vi "GetAndWriteSlowCtrl.vi"(0 "queue in":T11, 1 "notifier in":T10, 2 "Data In":T1={"DAQ Config Data"={"Vertical"={"Coupling"=1, "Offset (V)"=-0.5, "Range (V)"=2.0, "Impedance"=50.0}, "Horizontal"={"Offset Time"=0.0, "Sample Time (S)"=22.0, "Sample Points"=1000}, "Trigger\n"={"Lower Level (V)"=-0.02, "Trigger Slope"=1, "Trigger Source"=10}, "Acquisition"={"Trigger Mode"=1, "Initiate Continuously"=0, "Acquire Type"=0, "Acquire Count"=1}, "Channel"=0, "Instrument Handle"=0, "Error"={"status"=FALSE, "code"=0, "source"=""}, "State"=1}, "Acquisition"={"Current"={"Acquiring Now?"=FALSE, "Waveforms Acquired"=0.0, "Start of Acquisition"=timestamp(0 s since 1904-01-01), "Acquisition Name"=""}, "Stop Condition"={"Quota"=3000.0, "Duration (S)"=22, "Stop Condition"=FALSE}, "Config Needed"=FALSE}, "Measurement"={"Waveform"={"t0"=timestamp(0 s since 1904-01-01), "dt"=1.0, "Y"=[]}, "Peak Heights"=[], "Acquisition Time"=timestamp(0 s since 1904-01-01), "File Path"=path "C:/Users/lab-341/Desktop/Reed/Oscilloscope VI/pulses.tdms", "TDMS File Handle"=refnum}, "UI References"={"Acquire"=refnum, "Configure DAQ"=refnum, "Measurement (Ch1)"=refnum, "Update Needed?"=FALSE, "New Run"=refnum, "Signal"=refnum}, "Run Info"={"Active Run?"=FALSE, "Run Notes"="Enter in notes explaining the purpose of the run and any unusual steps taken in the process. This should make it clear why the data was taken. e.g. \"Measuring LXe scintillation light with Teflon\" or \"Measuring dark pulses to determine SPE gain.\" Concise is good but precise is better.", "User Name"="", "Campaign ID#"="", "Run Name"="", "Start Time"=timestamp(0 s since 1904-01-01), "End Time"=timestamp(0 s since 1904-01-01)}, "System Status"={"Bias Voltage"=0.0, "SiPM Temperature"=[], "Slow Control User"="", "LXe"=0.0}, "Acquisition Info"={"Trigger Mode"=FALSE, "Acquisition Mode"=FALSE, "Bias Voltage (V)"=0.0, "Preamplifier"=0, "Shaping Amplifier"=0, "Acquisition Notes"="", "1"=FALSE, "2"=FALSE}} {"Acquisition Info"."Shaping Amplifier" items=["CR-200-100ns", "CR-200-1us"]; "Acquisition Info"."Preamplifier" items=["CR-Z-113-1k", "CR-Z-113-5k", "CR-Z-SiPM"]; "DAQ Config Data"."State" items=["Enable"=1, "Disable"=0]; "DAQ Config Data"."Channel" items=["Input Channel 1", "Input Channel 2", "Input Channel 3", "Input Channel 4"]; "DAQ Config Data"."Acquisition"."Acquire Type" items=["Normal"=0, "Average"=1, "Envelope"=2, "Peak Detect"=3, "High Resolution"=4, "Fast"=5, "Equivalent Time"=16]; "DAQ Config Data"."Acquisition"."Initiate Continuously" items=["Continuously"=1, "Single Capture"=0]; "DAQ Config Data"."Acquisition"."Trigger Mode" items=["Auto", "Normal"]; "DAQ Config Data"."Trigger"."Trigger Source" items=["TTL0", "TTL1", "TTL2", "TTL3", "TTL4", "TTL5", "TTL6", "TTL7", "ECL0", "ECL1", "Input Channel 1", "Input Channel 2", "Input Channel 3", "Input Channel 4", "External Trigger Source", "STAR", "Manual Trigger", "Pattern"]; "DAQ Config Data"."Trigger"."Trigger Slope" items=["Rising Edge", "Falling Edge"]; "DAQ Config Data"."Horizontal"."Sample Time (S)" items=["0.5"=0.5, "0.4"=0.4, "0.25"=0.25, "0.2"=0.2, "0.1"=0.1, "0.05"=0.05, "0.04"=0.04, "0.025"=0.025, "0.02"=0.02, "0.01"=0.01, "0.005"=0.005, "0.004"=0.004, "0.0025"=0.0025, "0.002"=0.002, "0.001"=0.001, "5E-4"=0.0005, "4E-4"=0.0004, "2.5E-4"=0.00025, "2E-4"=0.0002, "1E-4"=0.0001, "5E-5"=5e-05, "4E-5"=4e-05, "2E-5"=2e-05, "5E-6"=5e-06, "1E-6"=1e-06, "5E-7"=5e-07, "1E-7"=1e-07, "5E-8"=5e-08, "1E-8"=1e-08]; "DAQ Config Data"."Vertical"."Impedance" items=["50 Ohm"=50.0, "1 MOhm"=1000000.0]; "DAQ Config Data"."Vertical"."Range (V)" items=["10"=10.0, "5"=5.0, "2"=2.0, "1"=1.0, "0.4"=0.4, "0.2"=0.2, "0.08"=0.08, "0.04"=0.04, "0.02"=0.02, "0.01"=0.01]; "DAQ Config Data"."Vertical"."Coupling" items=["AC", "DC"]}) -> (7 "queue out":T11, 8 "notifier out":T10, 9 "Data Out":T1={"DAQ Config Data"={"Vertical"={"Coupling"=1, "Offset (V)"=-0.5, "Range (V)"=2.0, "Impedance"=50.0}, "Horizontal"={"Offset Time"=0.0, "Sample Time (S)"=22.0, "Sample Points"=1000}, "Trigger\n"={"Lower Level (V)"=-0.02, "Trigger Slope"=1, "Trigger Source"=10}, "Acquisition"={"Trigger Mode"=1, "Initiate Continuously"=0, "Acquire Type"=0, "Acquire Count"=1}, "Channel"=0, "Instrument Handle"=0, "Error"={"status"=FALSE, "code"=0, "source"=""}, "State"=1}, "Acquisition"={"Current"={"Acquiring Now?"=FALSE, "Waveforms Acquired"=0.0, "Start of Acquisition"=timestamp(0 s since 1904-01-01), "Acquisition Name"=""}, "Stop Condition"={"Quota"=3000.0, "Duration (S)"=22, "Stop Condition"=FALSE}, "Config Needed"=FALSE}, "Measurement"={"Waveform"={"t0"=timestamp(0 s since 1904-01-01), "dt"=1.0, "Y"=[]}, "Peak Heights"=[], "Acquisition Time"=timestamp(0 s since 1904-01-01), "File Path"=path "C:/Users/lab-341/Desktop/Reed/Oscilloscope VI/pulses.tdms", "TDMS File Handle"=refnum}, "UI References"={"Acquire"=refnum, "Configure DAQ"=refnum, "Measurement (Ch1)"=refnum, "Update Needed?"=FALSE, "New Run"=refnum, "Signal"=refnum}, "Run Info"={"Active Run?"=FALSE, "Run Notes"="Enter in notes explaining the purpose of the run and any unusual steps taken in the process. This should make it clear why the data was taken. e.g. \"Measuring LXe scintillation light with Teflon\" or \"Measuring dark pulses to determine SPE gain.\" Concise is good but precise is better.", "User Name"="", "Campaign ID#"="", "Run Name"="", "Start Time"=timestamp(0 s since 1904-01-01), "End Time"=timestamp(0 s since 1904-01-01)}, "System Status"={"Bias Voltage"=0.0, "SiPM Temperature"=[], "Slow Control User"="", "LXe"=0.0}, "Acquisition Info"={"Trigger Mode"=FALSE, "Acquisition Mode"=FALSE, "Bias Voltage (V)"=0.0, "Preamplifier"=0, "Shaping Amplifier"=0, "Acquisition Notes"="", "1"=FALSE, "2"=FALSE}} {"Acquisition Info"."Shaping Amplifier" items=["CR-200-100ns", "CR-200-1us"]; "Acquisition Info"."Preamplifier" items=["CR-Z-113-1k", "CR-Z-113-5k", "CR-Z-SiPM"]; "DAQ Config Data"."State" items=["Enable"=1, "Disable"=0]; "DAQ Config Data"."Channel" items=["Input Channel 1", "Input Channel 2", "Input Channel 3", "Input Channel 4"]; "DAQ Config Data"."Acquisition"."Acquire Type" items=["Normal"=0, "Average"=1, "Envelope"=2, "Peak Detect"=3, "High Resolution"=4, "Fast"=5, "Equivalent Time"=16]; "DAQ Config Data"."Acquisition"."Initiate Continuously" items=["Continuously"=1, "Single Capture"=0]; "DAQ Config Data"."Acquisition"."Trigger Mode" items=["Auto", "Normal"]; "DAQ Config Data"."Trigger"."Trigger Source" items=["TTL0", "TTL1", "TTL2", "TTL3", "TTL4", "TTL5", "TTL6", "TTL7", "ECL0", "ECL1", "Input Channel 1", "Input Channel 2", "Input Channel 3", "Input Channel 4", "External Trigger Source", "STAR", "Manual Trigger", "Pattern"]; "DAQ Config Data"."Trigger"."Trigger Slope" items=["Rising Edge", "Falling Edge"]; "DAQ Config Data"."Horizontal"."Sample Time (S)" items=["0.5"=0.5, "0.4"=0.4, "0.25"=0.25, "0.2"=0.2, "0.1"=0.1, "0.05"=0.05, "0.04"=0.04, "0.025"=0.025, "0.02"=0.02, "0.01"=0.01, "0.005"=0.005, "0.004"=0.004, "0.0025"=0.0025, "0.002"=0.002, "0.001"=0.001, "5E-4"=0.0005, "4E-4"=0.0004, "2.5E-4"=0.00025, "2E-4"=0.0002, "1E-4"=0.0001, "5E-5"=5e-05, "4E-5"=4e-05, "2E-5"=2e-05, "5E-6"=5e-06, "1E-6"=1e-06, "5E-7"=5e-07, "1E-7"=1e-07, "5E-8"=5e-08, "1E-8"=1e-08]; "DAQ Config Data"."Vertical"."Impedance" items=["50 Ohm"=50.0, "1 MOhm"=1000000.0]; "DAQ Config Data"."Vertical"."Range (V)" items=["10"=10.0, "5"=5.0, "2"=2.0, "1"=1.0, "0.4"=0.4, "0.2"=0.2, "0.08"=0.08, "0.04"=0.04, "0.02"=0.02, "0.01"=0.01]; "DAQ Config Data"."Vertical"."Coupling" items=["AC", "DC"]})   [LabVIEW 2023]
uses:
  TypeDefs/DataTypes/Data.ctl
  TypeDefs/DataTypes/DAQConfig.ctl
  TypeDefs/DataTypes/Acquisition.ctl
  TypeDefs/DataTypes/Current.ctl
  TypeDefs/DataTypes/StopCondition.ctl
  TypeDefs/DataTypes/Measurement.ctl
  TypeDefs/DataTypes/UIReferences.ctl
  TypeDefs/DataTypes/RunInfo.ctl
  TypeDefs/DataTypes/SystemStatus.ctl
  TypeDefs/QueueNotifier/Notifier.ctl
  TypeDefs/QueueNotifier/DataQueue.ctl
  <vilib>/addons/h5labview2/file/H5Fmode.ctl
  <vilib>/addons/h5labview2/base/lib_path.vi
  <vilib>/addons/h5labview2/base/H5Equery.vi
  <vilib>/addons/h5labview2/attrib/H5Awrite.llb/H5Awrite.xnode
  <vilib>/Analysis/NI_AALBase.lvlib
  <vilib>/addons/h5labview2/file/H5F.lvlib
  <vilib>/addons/h5labview2/group/H5G.lvlib
panel:
  # "Shaper Gain"
  # "Self"
  # "Fast"
  # "Solicited"
  # "Standard"
  # "Shaper Gain"
  # "Self"
  # "Fast"
  # "Solicited"
  # "Standard"
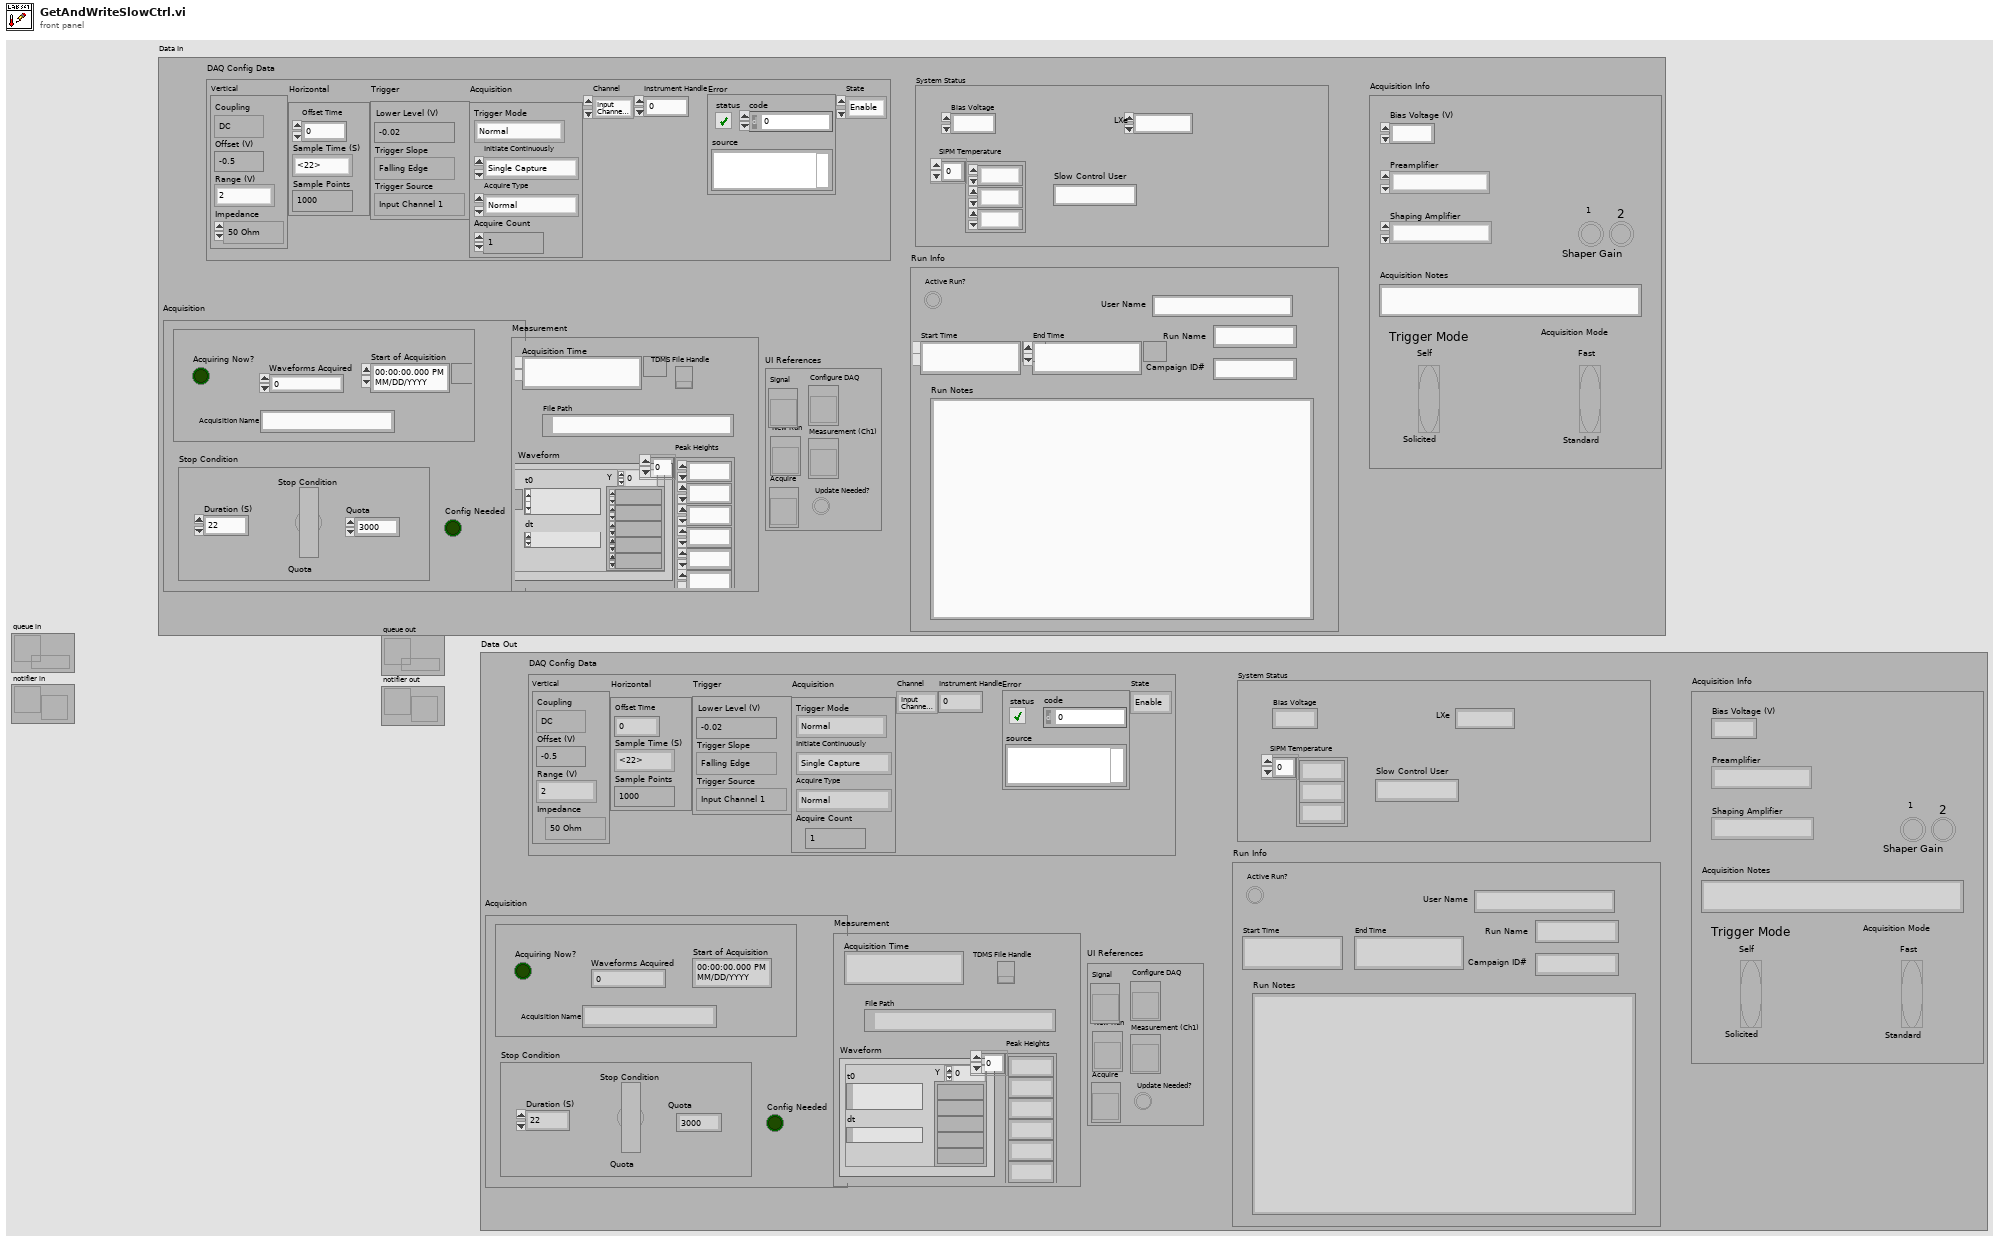
[diagram p1: front panel]
types:
  T1 = typedef "Data.ctl" = cluster{"DAQ Config Data":T2, "Acquisition":T3, "Measurement":T6, "UI References":T7, "Run Info":T8, "System Status":T9, "Acquisition Info":cluster{"Trigger Mode":bool, "Acquisition Mode":bool, "Bias Voltage (V)":dbl, "Preamplifier":u16, "Shaping Amplifier":u16, "Acquisition Notes":string, "1":bool, "2":bool}}
  T2 = typedef "DAQConfig.ctl" = cluster{"Vertical":cluster{"Coupling":i32, "Offset (V)":dbl, "Range (V)":dbl, "Impedance":dbl}, "Horizontal":cluster{"Offset Time":dbl, "Sample Time (S)":dbl, "Sample Points":u32}, "Trigger\n":cluster{"Lower Level (V)":dbl, "Trigger Slope":i32, "Trigger Source":i32}, "Acquisition":cluster{"Trigger Mode":i32, "Initiate Continuously":i32, "Acquire Type":i32, "Acquire Count":i32}, "Channel":i32, "Instrument Handle":i32, "Error":errorcluster, "State":i32}
  T3 = typedef "Acquisition.ctl" = cluster{"Current":T4, "Stop Condition":T5, "Config Needed":bool}
  T4 = typedef "Current.ctl" = cluster{"Acquiring Now?":bool, "Waveforms Acquired":dbl, "Start of Acquisition":timestamp, "Acquisition Name":string}
  T5 = typedef "StopCondition.ctl" = cluster{"Quota":dbl, "Duration (S)":u16, "Stop Condition":bool}
  T6 = typedef "Measurement.ctl" = cluster{"Waveform":waveform(dbl), "Peak Heights":dbl[], "Acquisition Time":timestamp, "File Path":path, "TDMS File Handle":refnum<k34>}
  T7 = typedef "UIReferences.ctl" = cluster{"Acquire":refnum<vi>, "Configure DAQ":refnum<vi>, "Measurement (Ch1)":refnum<vi>, "Update Needed?":bool, "New Run":refnum<vi>, "Signal":refnum<vi>}
  T8 = typedef "RunInfo.ctl" = cluster{"Active Run?":bool, "Run Notes":string, "User Name":string, "Campaign ID#":string, "Run Name":string, "Start Time":timestamp, "End Time":timestamp}
  T9 = typedef "SystemStatus.ctl" = cluster{"Bias Voltage":dbl, "SiPM Temperature":dbl[], "Slow Control User":string, "LXe":dbl}
  T10 = typedef "Notifier.ctl" = refnum<notifier>
  T11 = typedef "DataQueue.ctl" = refnum<queue>
  T12 = typedef "H5F.lvlib/H5Fmode.ctl" = enum16{"read-only", "read-write", "overwrite", "create new", "open or create"}
  T13 = typedef "hid_t.ctl" = i64
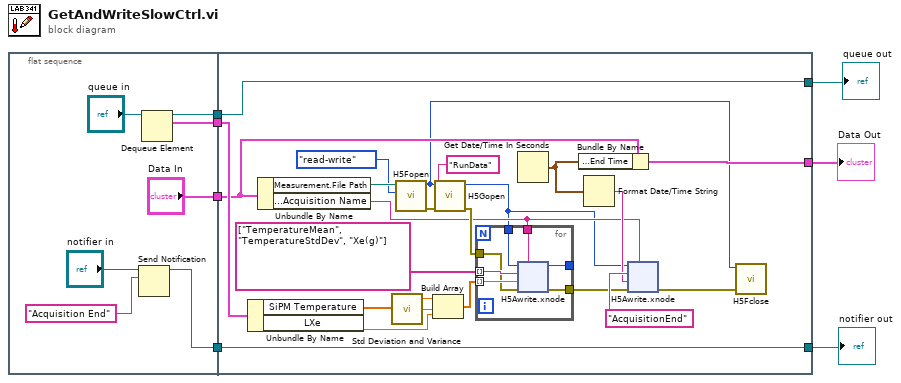
[diagram p0: block diagram]
diagram:
  n1 = flat-sequence {
    tunnel: [w12] -> w7
    tunnel: [w11] -> w3
    tunnel: [w10] -> w2
    tunnel: ["Data In"] -> w1
    tunnel: [w28] -> w5
    tunnel: w7 -> [w35]
    tunnel: [w35] -> w6
    tunnel: [w34] -> w4
    tunnel: w3 -> [w28]
    tunnel: w2 -> [w27]
    tunnel: w1 -> [w26]
    frame #0 {
      n2 = Send Notification(notification="Acquisition End", notifier="notifier in") -> (notifier out=w12:T10)  [unwired: 1 in, 1 out]
      n3 = Dequeue Element(queue="queue in") -> (queue out=w11:T11, element=w10:T9)  [unwired: 2 in, 2 out]
    }
    frame #1 {
      n4 = Unbundle By Name(w27) -> ("SiPM Temperature"=w38:dbl[], "LXe"=w16:dbl)
      n5 = Unbundle By Name(w26) -> ("Measurement.File Path"=w25:path, "Acquisition.Current.Acquisition Name"=w20:string)
      n6 = call <vilib>:"Std Deviation and Variance.vi"("X"=w38) -> ("mean"=w37:dbl, "standard deviation"=w36:dbl)  [unwired: 1 in, 1 out]
      n7 = call <vilib>:"H5Fopen.vi"("mode (read-only)"=H5Fmode."read-write", "path"=w25) -> ("error out"=w24:errorcluster, "ref out"=w19:T13)  [unwired: 8 in]
      n8 = Build Array(w37, w36, w16) -> (w31:dbl[])
      n9 = call <vilib>:"H5Gopen.vi"("error in (no error)"=w24, "name"="RunData", "ref in"=w19) -> ("error out"=w23:errorcluster, "group out"=w18:T13)  [unwired: 7 in]
      n10 = for {
        tunnel: string[] ["TemperatureMean", "TemperatureStdDev", "Xe(g)"] ("property names") -> [w64] mode=indexing
        tunnel: w31 -> [w63] mode=indexing
        tunnel: [w62] -> _
        tunnel: w18 -> [w61]
        tunnel: w23 -> [w60]
        tunnel: [w59] -> w22
        tunnel: w20 -> [w58]
        n11 = xnode "H5Awrite.xnode"("object name"=w58, "error in (no error)"=w60, "data"=w63, "attrib name"=w64, "ref in"=w61) -> ("error out"=w59:errorcluster, "ref out"=w62:i64)  [unwired: 2 in, 1 out]
      }
      n12 = Get Date/Time In Seconds() -> (seconds since 1Jan1904=w33:timestamp)
      n13 = Bundle By Name(cluster=w26, "Run Info.End Time"=w33) -> (w34:T1)
      n14 = Format Date/Time String(seconds (now)=w33) -> (date/time string=w29:string)  [unwired: 2 in]
      n15 = xnode "H5Awrite.xnode"("object name"=w20, "error in (no error)"=w22, "data"=w29, "attrib name"="AcquisitionEnd" ("property names"), "ref in"=w18) -> ("error out"=w15:errorcluster)  [unwired: 2 in, 2 out]
      n16 = call <vilib>:"H5Fclose.vi"("error in (no error)"=w15, "ref"=w19) -> ()  [unwired: 9 in, 1 out]
    }
  }
  "notifier out" <- w6
  "queue out" <- w5
  "Data Out" <- w4
